vi "SSL_Connect.vi"(8 "error in (no error)":errorcluster, 10 "SSL_Connection":T1, 11 "login":T2={"server IP"="", "server port"=0, "local port (0 = auto)"=0, "timeout ms (1000)"=1000}) -> (0 "error out":errorcluster, 2 "SSL_Connection":T1)   [LabVIEW 2015, in "AWS_IoT.lvlib"]
uses:
  AWS_IoT.lvlib
  Controls/SSL_login.ctl
  Controls/SSL_Connection.ctl
  <vilib>/httpClient/LabVIEWHTTPClient.lvlib
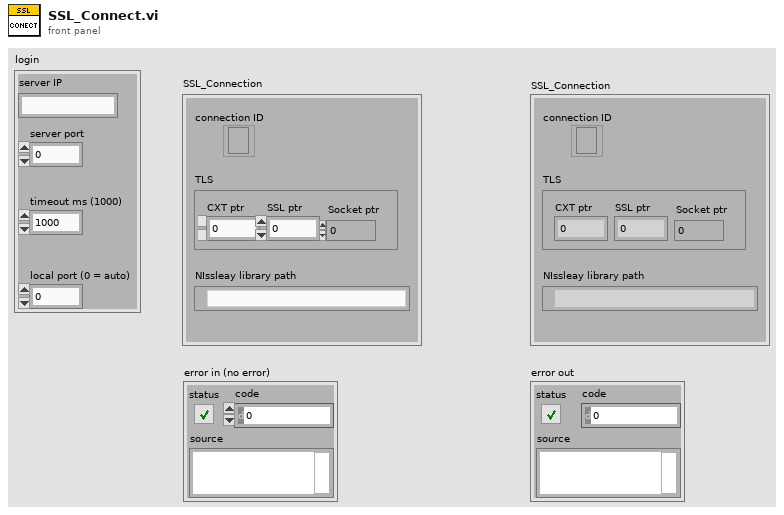
[diagram p1: front panel]
types:
  T1 = typedef "AWS_IoT.lvlib/SSL_Connection.ctl" = cluster{"connection ID":refnum<k5>, "TLS":cluster{"CXT ptr":i32, "SSL ptr":i32, "Socket ptr":u64}, "NIssleay library path":path}
  T2 = typedef "AWS_IoT.lvlib/SSL_login.ctl" = cluster{"server IP":string, "server port":u16, "local port (0 = auto)":u16, "timeout ms (1000)":i32}
  T3 = typedef "LabVIEWHTTPClient.lvlib/ClientHandle.ctl" = refnum<k1>
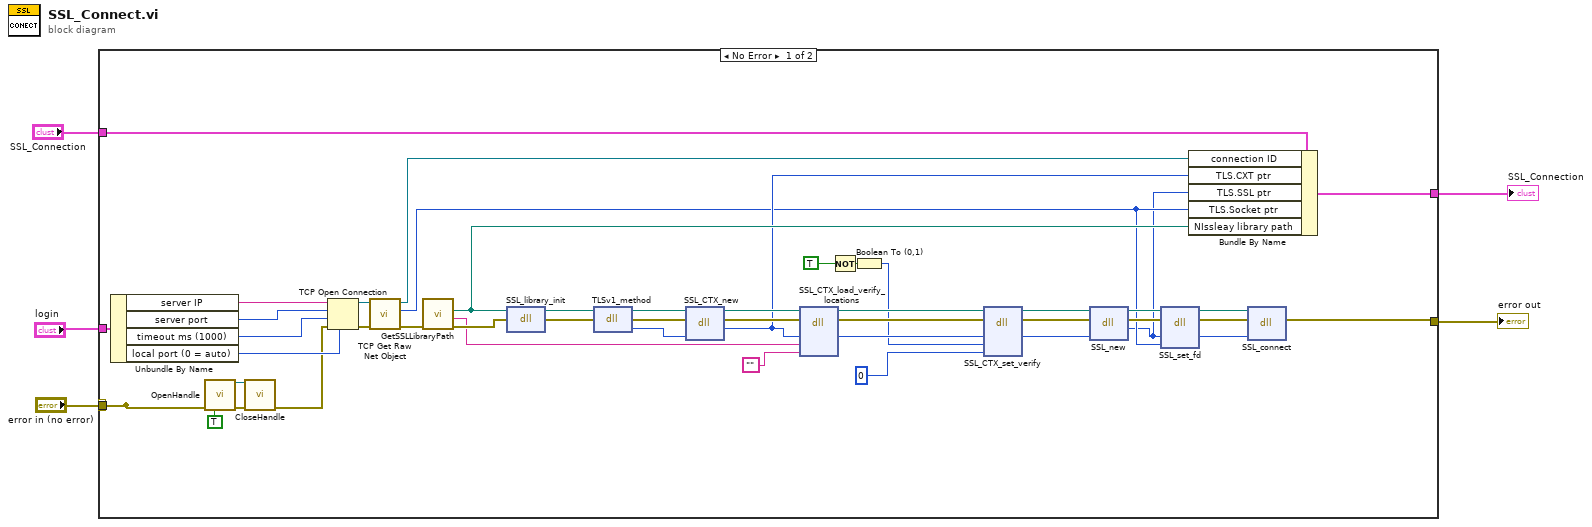
[diagram p0: block diagram]
diagram:
  n1 = case shown="No Error" "error in (no error)" {
    selector: "error in (no error)" -> [w8 w52]
    tunnel: "login" -> [w45 _]
    tunnel: "SSL_Connection" -> [w44 w53]
    tunnel: [w12 w53] -> w3
    tunnel: [w8 _] -> _
    tunnel: [w11 w52] -> w2
    frame No Error {
      n2 = Unbundle By Name(w45) -> ("server IP"=w49:string, "server port"=w48:u16, "timeout ms (1000)"=w47:i32, "local port (0 = auto)"=w46:u16)
      n3 = call <vilib>:"OpenHandle.vi"("error in (no error)"=w8, "verify server(true)"=TRUE) -> ("client handle out"=w10:T3, "error out"=w9:errorcluster)  [unwired: 12 in]
      n4 = call <vilib>:"CloseHandle.vi"("client handle"=w10, "error in (no error)"=w9) -> ("error out"=w7:errorcluster)  [unwired: 13 in]
      n5 = TCP Open Connection(address=w49, remote port or service name=w48, timeout ms (60000)=w47, local port=w46, error in (no error)=w7) -> (connection ID=w51:refnum<k5>, error out=w50:errorcluster)
      n6 = call <vilib>:"TCP Get Raw Net Object.vi"("error in (no error)"=w50, "connection ID"=w51) -> ("error out"=w25:errorcluster, "raw net object"=w20:u64, "connection ID out"=w43:refnum<k5>)  [unwired: 7 in]
      n7 = call "GetSSLLibraryPath.vi"("error in (no error)"=w25) -> ("error out"=w23:errorcluster, "CA-bundle.crt"=w22:string, "NIssleay library path"=w24:path)  [unwired: 7 in, 1 out]
      n8 = dll-call lib="NIssleay32.*" fn="SSL_library_init"(path in=w24, error in=w23) -> (path out=w31:path, error out=w26:errorcluster)  [unwired: 2 in]
      n9 = dll-call lib="NIssleay32.*" fn="TLSv1_method"(path in=w31, error in=w26) -> (path out=w32:path, error out=w27:errorcluster, "return type"=w28:i32)  [unwired: 1 in]
      n10 = dll-call lib="NIssleay32.*" fn="SSL_CTX_new"(path in=w32, error in=w27, "ClientMethod"=w28) -> (path out=w41:path, error out=w39:errorcluster, "return type"=w21:i32)  [unwired: 2 in]
      n11 = dll-call lib="NIssleay32.*" fn="SSL_CTX_load_verify_locations"(path in=w41, error in=w39, "CTX"=w21, "CAfile"=w22, "CApath"="") -> (path out=w42:path, error out=w40:errorcluster, "CTX"=w37:i32)  [unwired: 4 in]
      n12 = Not(x=TRUE) -> (.not. x?=w18:bool)
      n13 = Boolean To (0,1)(Boolean=w18) -> (0, 1=w16:i16)
      n14 = dll-call lib="NIssleay32.*" fn="SSL_CTX_set_verify"(path in=w42, error in=w40, "CTX"=w37, "mode"=w16, "verify_callback"=0) -> (path out=w33:path, error out=w34:errorcluster, "CTX"=w35:i32)  [unwired: 4 in]
      n15 = dll-call lib="NIssleay32.*" fn="SSL_new"(path in=w33, error in=w34, "Context"=w35) -> (path out=w29:path, error out=w30:errorcluster, "return type"=w19:i32)  [unwired: 2 in]
      n16 = dll-call lib="NIssleay32.*" fn="SSL_set_fd"(path in=w29, error in=w30, "SSL"=w19, "Socket"=w20) -> (path out=w15:path, error out=w14:errorcluster, "SSL"=w13:i32)  [unwired: 3 in]
      n17 = Bundle By Name(cluster=w44, "connection ID"=w43, "TLS.CXT ptr"=w21, "TLS.SSL ptr"=w19, "TLS.Socket ptr"=w20, "NIssleay library path"=w24) -> (w12:T1)
      n18 = dll-call lib="NIssleay32.*" fn="SSL_connect"(path in=w15, error in=w14, "SSL"=w13) -> (error out=w11:errorcluster)  [unwired: 3 in, 1 out]
    }
    frame Error {
    }
  }
  "SSL_Connection" <- w3
  "error out" <- w2
